vi "Sequence.Break.Check.vi"(10 "Pauses B":T2[](array[typedef]), 11 "Pauses A":T2[](array[typedef])) -> (1 "break source":T1, 2 "break reason":T2, 3 "break found":bool)   [LabVIEW 2016]
uses:
  Sequence.Test.BreakReason.ctl
  Sequence.Test.BreakSource.ctl
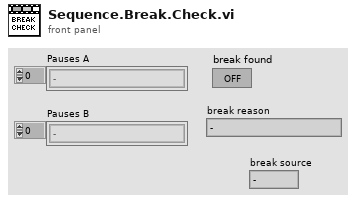
[diagram p1: front panel]
types:
  T1 = typedef "Sequence.Test.BreakSource.ctl" = enum16{"-", "A", "B", "A/B"}
  T2 = typedef "Sequence.Test.BreakReason.ctl" = enum16{"-", "NOK container", "OK container", "Rev empty", "Rev missing", "Rev wrong", "Fork missing", "Fork wrong", "NOK limit", "Unload failure", "Single slot", "Part done", "Err: Prod move work", "Err: Prod move home", "Err: Prod lift work", "Err: Prod lift home", "Err: Prod Arm Work", "Err: Prod Arm NOK", "Err: Prod Arm OK", "Err: Prod NOK suck", "Err: Prod NOK drop", "Err: Prod OK missing", "Err: Prod OK suck", "Err: Prod OK drop"}
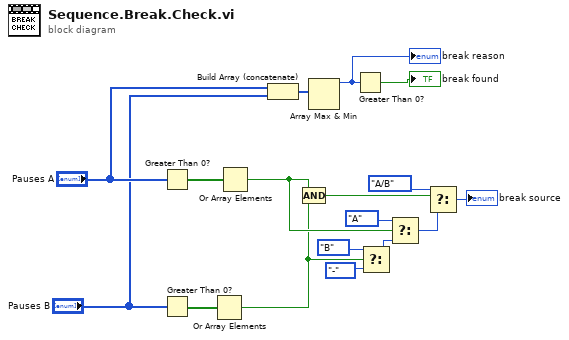
[diagram p0: block diagram]
diagram:
  n1 = Greater Than 0?(x="Pauses A") -> (x > 0?=w17:bool[])
  n2 = Greater Than 0?(x="Pauses B") -> (x > 0?=w11:bool[])
  n3 = Or Array Elements(Boolean array=w11) -> (logical OR=w5:bool)
  n4 = Or Array Elements(Boolean array=w17) -> (logical OR=w8:bool)
  n5 = Build Array (concatenate)("Pauses A", "Pauses B") -> (w16:T2[])
  n6 = Compound Arithmetic op=AND(w8, w5) -> (w10:bool)
  n7 = Array Max & Min(array=w16) -> (max value=w15:T2)  [unwired: 3 out]
  "break reason" <- w15
  n8 = Greater Than 0?(x=w15) -> (x > 0?=→"break found":bool)
  n9 = Select(t=Sequence.Test.BreakSource."B" ("break source"), s=w5, f=Sequence.Test.BreakSource."-" ("break source")) -> (s? t:f=w4:T1)
  n10 = Select(t=Sequence.Test.BreakSource."A" ("break source"), s=w8, f=w4) -> (s? t:f=w3:T1)
  n11 = Select(t=Sequence.Test.BreakSource."A/B" ("break source"), s=w10, f=w3) -> (s? t:f=→"break source":T1)
